vi "ArmNetwork.vi"(8 "error in (no error)":errorcluster) -> (0 "error out":errorcluster)   [LabVIEW 2020]
doc: "Network for Arm\n\nInputs:\n -- error in -- cluster\n\nOutputs:\n -- error in -- cluster"
uses:
  ArmGlobal.vi
  <vilib>/Rock Robotics/Network Tables/NT Write Number.vi
  <vilib>/Rock Robotics/Network Tables/NT Write Boolean.vi
  <vilib>/Rock Robotics/Network Tables/NT Write String.vi
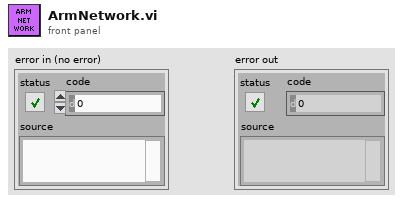
[diagram p1: front panel]
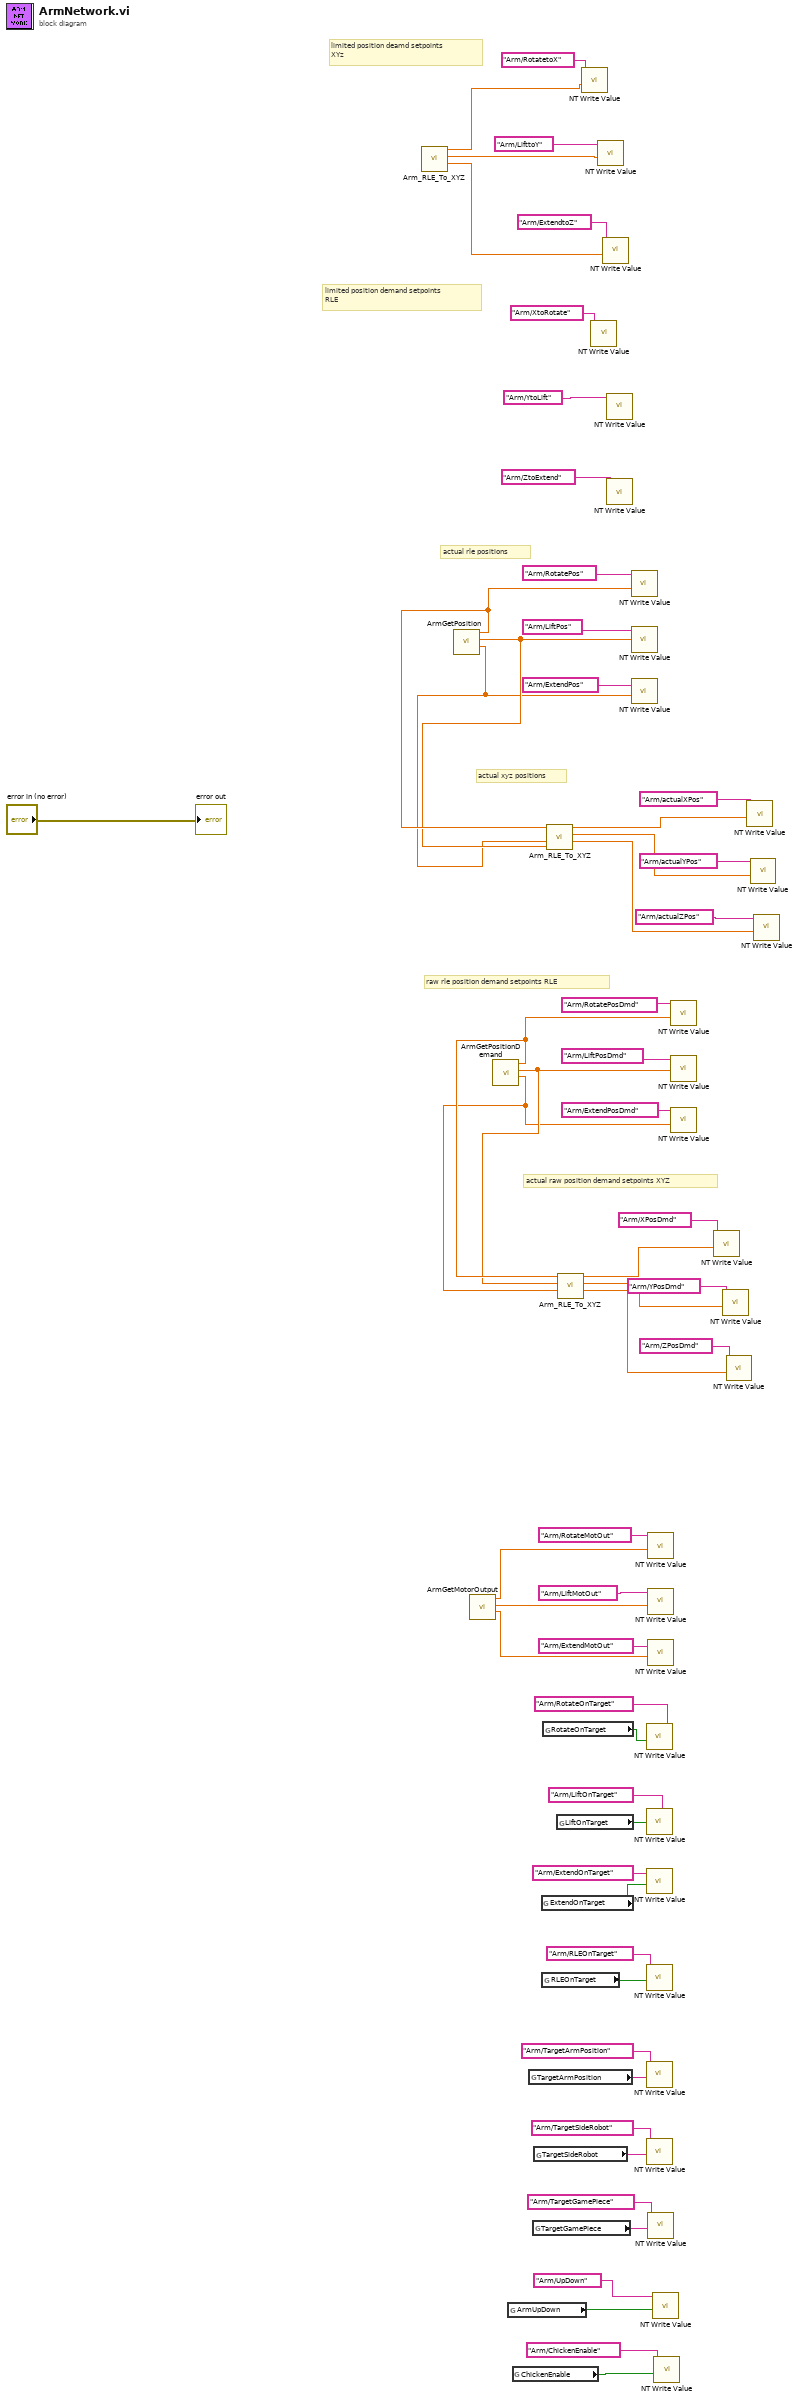
[diagram p0: block diagram]
diagram:
  # "actual xyz positions"
  # "actual raw position demand setpoints XYZ"
  # "limited position deamd setpoints\nXYz"
  # "limited position demand setpoints\nRLE"
  # "actual rle positions"
  # "raw rle position demand setpoints RLE"
  n1 = call "Arm_RLE_To_XYZ.vi"() -> ("z"=w19:dbl, "y"=w20:dbl, "x"=w21:dbl)  [unwired: 9 in]
  n2 = call "ArmGetPosition.vi"() -> ("ExtendPostion"=w10:dbl, "LiftPostion"=w17:dbl, "RotatePostion"=w18:dbl)  [unwired: 9 in]
  n3 = call "ArmGetMotorOutput.vi"() -> ("ExtendMotorOutput"=w55:dbl, "LiftMotorOutput"=w56:dbl, "RotateMotorOutput"=w57:dbl)  [unwired: 9 in]
  n4 = call "ArmGetPositionDemand.vi"() -> ("ExtendPositonDemand(in)"=w7:dbl, "LiftPositionDemand(d)"=w8:dbl, "RotatePositonDemand(d)"=w9:dbl)  [unwired: 9 in]
  n5 = global read "ArmGlobal.vi" "ArmUpDown"() -> (w31:bool)
  n6 = global read "ArmGlobal.vi" "ChickenEnable"() -> (w29:bool)
  n7 = global read "ArmGlobal.vi" "TargetArmPosition"() -> (w37:string)
  n8 = global read "ArmGlobal.vi" "TargetGamePiece"() -> (w33:string)
  n9 = global read "ArmGlobal.vi" "TargetSideRobot"() -> (w35:string)
  n10 = global read "ArmGlobal.vi" "ExtendOnTarget"() -> (w41:bool)
  n11 = global read "ArmGlobal.vi" "RLEOnTarget"() -> (w39:bool)
  n12 = global read "ArmGlobal.vi" "RotateOnTarget"() -> (w45:bool)
  n13 = call "Arm_RLE_To_XYZ.vi"("Extend"=w10, "Lift"=w17, "Rotate"=w18) -> ("z"=w14:dbl, "y"=w15:dbl, "x"=w16:dbl)  [unwired: 6 in]
  n14 = global read "ArmGlobal.vi" "LiftOnTarget"() -> (w44:bool)
  n15 = call "Arm_RLE_To_XYZ.vi"("Extend"=w7, "Lift"=w8, "Rotate"=w9) -> ("z"=w4:dbl, "y"=w5:dbl, "x"=w6:dbl)  [unwired: 6 in]
  n16 = call-poly <vilib>:"NT Write Value.vi"("value"=w21, "name"="Arm/RotatetoX") -> ()  [unwired: 9 in, 1 out]
  n17 = call-poly <vilib>:"NT Write Value.vi"("name"="Arm/XtoRotate") -> ()  [unwired: 10 in, 1 out]
  n18 = call-poly <vilib>:"NT Write Value.vi"("value"=w20, "name"="Arm/LifttoY") -> ()  [unwired: 9 in, 1 out]
  n19 = call-poly <vilib>:"NT Write Value.vi"("value"=w19, "name"="Arm/ExtendtoZ") -> ()  [unwired: 9 in, 1 out]
  n20 = call-poly <vilib>:"NT Write Value.vi"("name"="Arm/YtoLift") -> ()  [unwired: 10 in, 1 out]
  n21 = call-poly <vilib>:"NT Write Value.vi"("name"="Arm/ZtoExtend") -> ()  [unwired: 10 in, 1 out]
  n22 = call-poly <vilib>:"NT Write Value.vi"("value"=w18, "name"="Arm/RotatePos") -> ()  [unwired: 9 in, 1 out]
  n23 = call-poly <vilib>:"NT Write Value.vi"("value"=w17, "name"="Arm/LiftPos") -> ()  [unwired: 9 in, 1 out]
  n24 = call-poly <vilib>:"NT Write Value.vi"("value"=w10, "name"="Arm/ExtendPos") -> ()  [unwired: 9 in, 1 out]
  n25 = call-poly <vilib>:"NT Write Value.vi"("value"=w45, "name"="Arm/RotateOnTarget") -> ()  [unwired: 9 in, 1 out]
  n26 = call-poly <vilib>:"NT Write Value.vi"("value"=w44, "name"="Arm/LiftOnTarget") -> ()  [unwired: 9 in, 1 out]
  n27 = call-poly <vilib>:"NT Write Value.vi"("value"=w41, "name"="Arm/ExtendOnTarget") -> ()  [unwired: 9 in, 1 out]
  n28 = call-poly <vilib>:"NT Write Value.vi"("value"=w39, "name"="Arm/RLEOnTarget") -> ()  [unwired: 9 in, 1 out]
  n29 = call-poly <vilib>:"NT Write Value.vi"("value"=w37, "name"="Arm/TargetArmPosition") -> ()  [unwired: 9 in, 1 out]
  n30 = call-poly <vilib>:"NT Write Value.vi"("value"=w35, "name"="Arm/TargetSideRobot") -> ()  [unwired: 9 in, 1 out]
  n31 = call-poly <vilib>:"NT Write Value.vi"("value"=w57, "name"="Arm/RotateMotOut") -> ()  [unwired: 9 in, 1 out]
  n32 = call-poly <vilib>:"NT Write Value.vi"("value"=w56, "name"="Arm/LiftMotOut") -> ()  [unwired: 9 in, 1 out]
  n33 = call-poly <vilib>:"NT Write Value.vi"("value"=w55, "name"="Arm/ExtendMotOut") -> ()  [unwired: 9 in, 1 out]
  n34 = call-poly <vilib>:"NT Write Value.vi"("value"=w33, "name"="Arm/TargetGamePiece") -> ()  [unwired: 9 in, 1 out]
  n35 = call-poly <vilib>:"NT Write Value.vi"("value"=w31, "name"="Arm/UpDown") -> ()  [unwired: 9 in, 1 out]
  n36 = call-poly <vilib>:"NT Write Value.vi"("value"=w29, "name"="Arm/ChickenEnable") -> ()  [unwired: 9 in, 1 out]
  n37 = call-poly <vilib>:"NT Write Value.vi"("value"=w9, "name"="Arm/RotatePosDmd") -> ()  [unwired: 9 in, 1 out]
  n38 = call-poly <vilib>:"NT Write Value.vi"("value"=w8, "name"="Arm/LiftPosDmd") -> ()  [unwired: 9 in, 1 out]
  n39 = call-poly <vilib>:"NT Write Value.vi"("value"=w7, "name"="Arm/ExtendPosDmd") -> ()  [unwired: 9 in, 1 out]
  n40 = call-poly <vilib>:"NT Write Value.vi"("value"=w6, "name"="Arm/XPosDmd") -> ()  [unwired: 9 in, 1 out]
  n41 = call-poly <vilib>:"NT Write Value.vi"("value"=w5, "name"="Arm/YPosDmd") -> ()  [unwired: 9 in, 1 out]
  n42 = call-poly <vilib>:"NT Write Value.vi"("value"=w4, "name"="Arm/ZPosDmd") -> ()  [unwired: 9 in, 1 out]
  n43 = call-poly <vilib>:"NT Write Value.vi"("value"=w16, "name"="Arm/actualXPos") -> ()  [unwired: 9 in, 1 out]
  n44 = call-poly <vilib>:"NT Write Value.vi"("value"=w15, "name"="Arm/actualYPos") -> ()  [unwired: 9 in, 1 out]
  n45 = call-poly <vilib>:"NT Write Value.vi"("value"=w14, "name"="Arm/actualZPos") -> ()  [unwired: 9 in, 1 out]
  "error out" <- "error in (no error)"
